vi "Main.vi"() -> ()   [LabVIEW 2017]
panel:
  out "Displacement Array":dbl[](array[numeric])
  out "Velocty Array":dbl[](array[numeric])
  out "Accel Array":dbl[](array[numeric])
  out "Displacement":dbl[](graph)
  out "Velocity":dbl[](graph)
  out "Acceleration":dbl[](graph)
  out "Motion Planning Outputs":T1
  out "No limit speed (mm/s)":dbl
  in  "Motion Planning Inputs":T2
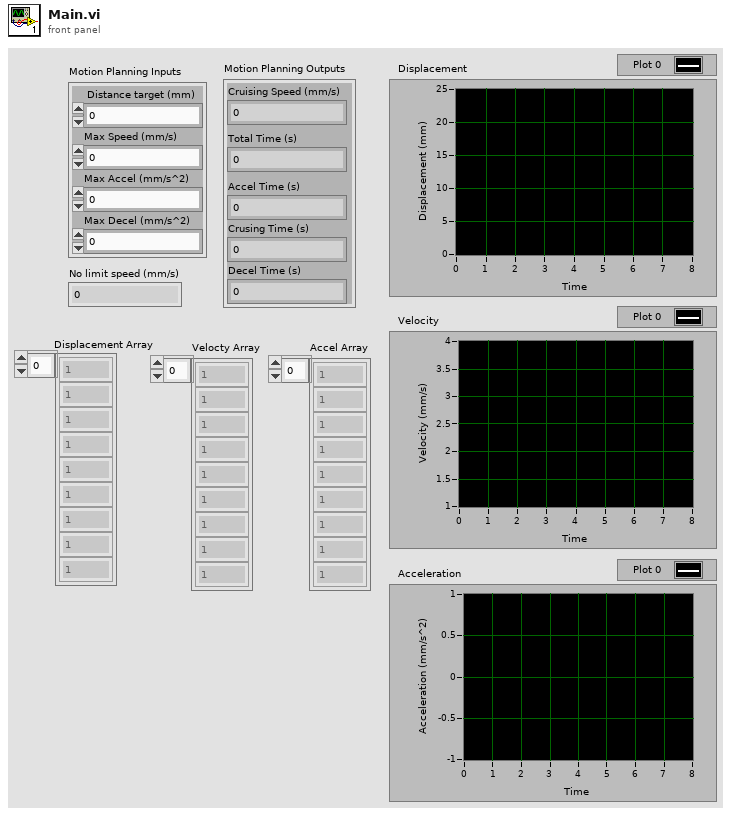
[diagram p1: front panel]
types:
  T1 = cluster{"Cruising Speed (mm/s)":dbl, "Crusing Time (s)":dbl, "Decel Time (s)":dbl, "Accel Time (s)":dbl, "Total Time (s)":dbl}
  T2 = cluster{" Distance target (mm)":dbl, "Max Accel (mm/s^2)":dbl, "Max Decel (mm/s^2)":dbl, "Max Speed (mm/s) ":dbl}
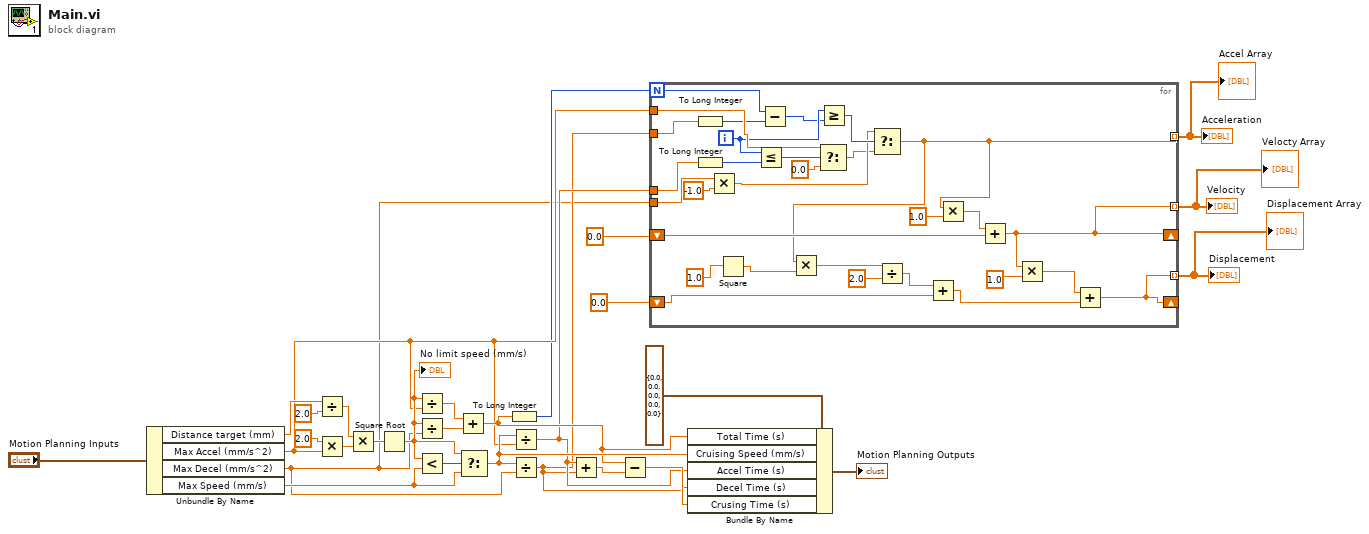
[diagram p0: block diagram]
diagram:
  n1 = Unbundle By Name("Motion Planning Inputs") -> ("Distance target (mm)"=w25:dbl, "Max Accel (mm/s^2)"=w9:dbl, "Max Decel (mm/s^2)"=w6:dbl, "Max Speed (mm/s)"=w20:dbl)
  n2 = Divide(x=w25, y=2.0) -> (x/y=w23:dbl)
  n3 = Multiply(x=2.0, y=w9) -> (x*y=w26:dbl)
  n4 = Multiply(x=w23, y=w26) -> (x*y=w13:dbl)
  n5 = Square Root(x=w13) -> (sqrt(x)=w12:dbl)
  "No limit speed (mm/s)" <- w12
  n6 = Divide(x=w12, y=w9) -> (x/y=w18:dbl)
  n7 = Divide(x=w12, y=w6) -> (x/y=w17:dbl)
  n8 = Less?(x=w12, y=w20) -> (x < y?=w22:bool)
  n9 = Add(x=w18, y=w17) -> (x+y=w11:dbl)
  n10 = Select(t=w12, s=w22, f=w20) -> (s? t:f=w16:dbl)
  n11 = To Long Integer(number=w11) -> (32bit integer=w8:i32)
  n12 = Divide(x=w16, y=w9) -> (x/y=w10:dbl)
  n13 = Divide(x=w16, y=w6) -> (x/y=w7:dbl)
  n14 = Add(x=w10, y=w7) -> (x+y=w14:dbl)
  n15 = Subtract(x=w11, y=w14) -> (x-y=w15:dbl)
  n16 = for {
    N: w8 -> [w53]
    tunnel: w10 -> [w58]
    tunnel: w9 -> [w54]
    tunnel: [w35] -> w3 mode=indexing
    tunnel: w7 -> [w52]
    tunnel: w6 -> [w48]
    shift-right: [w38] -> _
    shift-left: 0.0 -> [w43]
    tunnel: [w38] -> w2 mode=indexing
    shift-right: [w29] -> _
    shift-left: 0.0 -> [w31]
    tunnel: [w29] -> w1 mode=indexing
    i -> [w51]
    n17 = To Long Integer(number=w52) -> (32bit integer=w45:i32)
    n18 = To Long Integer(number=w58) -> (32bit integer=w57:i32)
    n19 = Multiply(x=w48, y=-1.0) -> (x*y=w46:dbl)
    n20 = Square(x=1.0 ("y")) -> (x^2=w36:dbl)
    n21 = Less Or Equal?(x=w51, y=w57) -> (x <= y?=w56:bool)
    n22 = Subtract(x=w53, y=w45) -> (x-y=w50:i32)
    n23 = Select(t=w54, s=w56, f=0.0) -> (s? t:f=w44:dbl)
    n24 = Greater Or Equal?(x=w51, y=w50) -> (x >= y?=w49:bool)
    n25 = Select(t=w46, s=w49, f=w44) -> (s? t:f=w35:dbl)
    n26 = Multiply(x=w35, y=w36) -> (x*y=w34:dbl)
    n27 = Divide(x=w34, y=2.0) -> (x/y=w32:dbl)
    n28 = Add(x=w32, y=w31) -> (x+y=w30:dbl)
    n29 = Multiply(x=w35, y=1.0) -> (x*y=w41:dbl)
    n30 = Add(x=w41, y=w43) -> (x+y=w38:dbl)
    n31 = Multiply(x=w38, y=1.0) -> (x*y=w39:dbl)
    n32 = Add(x=w39, y=w30) -> (x+y=w29:dbl)
  }
  "Acceleration" <- w3
  "Velocity" <- w2
  "Displacement" <- w1
  "Accel Array" <- w3
  "Velocty Array" <- w2
  "Displacement Array" <- w1
  n33 = Bundle By Name(cluster=T1 {"Cruising Speed (mm/s)"=0.0, "Crusing Time (s)"=0.0, "Decel Time (s)"=0.0, "Accel Time (s)"=0.0, "Total Time (s)"=0.0} ("Motion Planning Outputs"), "Total Time (s)"=w11, "Cruising Speed (mm/s)"=w16, "Accel Time (s)"=w10, "Decel Time (s)"=w7, "Crusing Time (s)"=w15) -> (→"Motion Planning Outputs":T1)
